vi "Insert Image.vi"(8 "error in (no error)":errorcluster, 11 "EmbedImage in":refnum<class "EmbedImage.lvclass">) -> (0 "error out":errorcluster, 3 "EmbedImage out":refnum<class "EmbedImage.lvclass">)   [LabVIEW 2023, in "EmbedImage.lvlib" / "EmbedImage.lvclass"]
uses:
  Library/EmbedImage.lvclass
  Library/EmbedImage.lvclass/EmbedImage.ctl
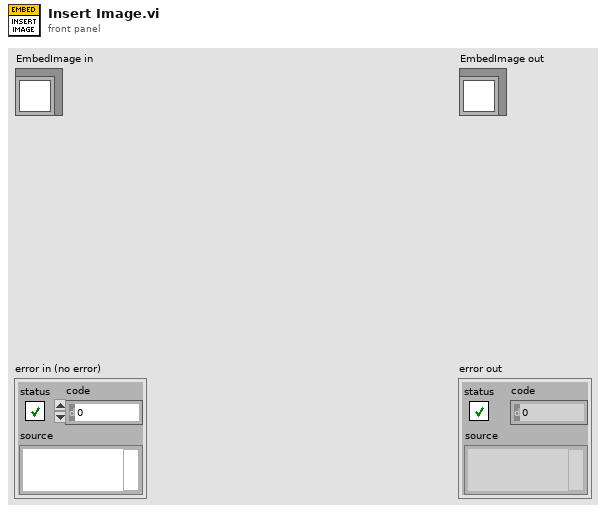
[diagram p1: front panel]
types:
  T1 = typedef "imagedata.ctl" = cluster{"image type":i32, "image depth":i32, "image":u8[], "mask":u8[], "colors":u32[], "Rectangle":cluster{"left":i16, "top":i16, "right":i16, "bottom":i16}}
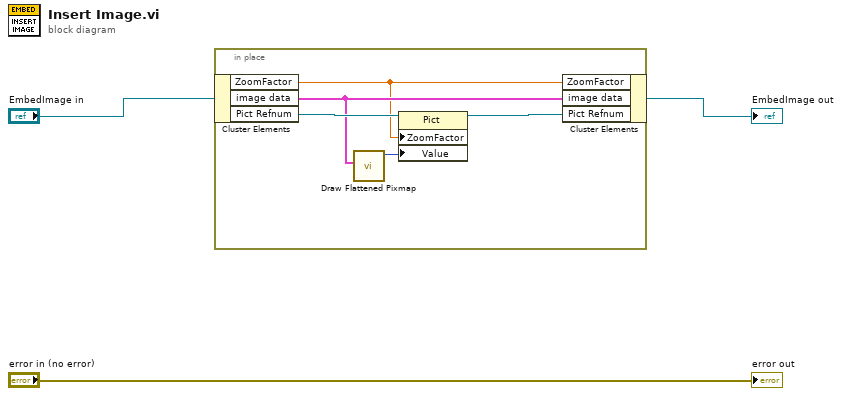
[diagram p0: block diagram]
diagram:
  n1 = in-place {
    n2 = in-place-cluster #1("EmbedImage in") -> ("ZoomFactor"=w4:dbl, "image data"=w6:T1, "Pict Refnum"=w8:refnum<vi>)
    n3 = call <vilib>:"Draw Flattened Pixmap.vi"("image data"=w6) -> ("new picture"=w5:picture)  [unwired: 8 in]
    n4 = property class="Pict"(reference=w8, "ZoomFactor"=w4, "Value"=w5) -> (reference out=w7:refnum<vi>)  [unwired: 1 in, 1 out]
    n5 = in-place-cluster #1("ZoomFactor"=w4, "image data"=w6, "Pict Refnum"=w7) -> (→"EmbedImage out":refnum<class "EmbedImage.lvclass">)
  }
  "error out" <- "error in (no error)"
